vi "prepare.vi"(8 "error in (no error)":errorcluster, 11 "Pizza in":refnum<class "Pizza.lvclass">) -> (0 "error out":errorcluster, 2 "preparing message":string, 3 "Pizza out":refnum<class "Pizza.lvclass">)   [LabVIEW 2021, in "Pizza.lvclass"]
uses:
  Pizza.lvclass
  Pizza.lvclass/Pizza.ctl
panel:
  # "Connector Pane"
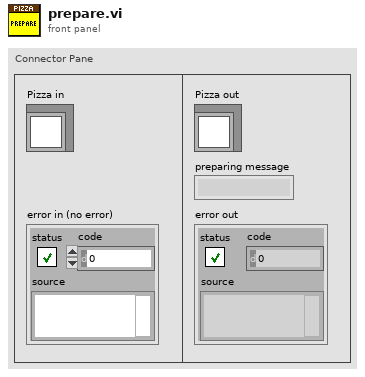
[diagram p1: front panel]
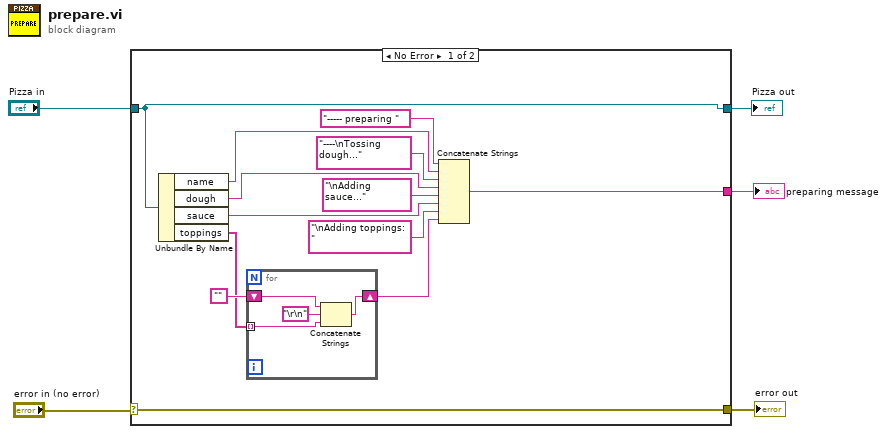
[diagram p0: block diagram]
diagram:
  n1 = case shown="No Error" "error in (no error)" {
    selector: "error in (no error)" -> [w18 w24]
    tunnel: [w18 w24] -> w4
    tunnel: [w17 w23] -> w2
    tunnel: "Pizza in" -> [w17 w23]
    tunnel: [w11 _] -> w1
    frame No Error {
      n2 = Unbundle By Name(w17) -> ("name"=w15:string, "dough"=w8:string, "sauce"=w6:string, "toppings"=w10:string[])
      n3 = for {
        tunnel: w10 -> [w19] mode=indexing
        shift-right: [w22] -> w12
        shift-left: "" -> [w21]
        n4 = Concatenate Strings(w21, "\r\n", w19) -> (w22:string)
      }
      n5 = Concatenate Strings("----- preparing ", w15, "----\nTossing dough..." ("string"), w8, "\nAdding sauce..." ("string"), w6, "\nAdding toppings: " ("string"), w12) -> (w11:string)
    }
    frame Error {
    }
  }
  "error out" <- w4
  "Pizza out" <- w2
  "preparing message" <- w1
